vi "first.vi"() -> ()   [LabVIEW 2019]
panel:
  in  "Boolean":bool
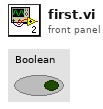
[diagram p1: front panel]
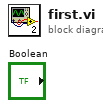
[diagram p0: block diagram]
diagram:
